vi "Get Next Round.vi"(11 "Square in":refnum<class "Square.lvclass">) -> (2 "Next Round":u32, 3 "Square out":refnum<class "Square.lvclass">)   [LabVIEW 2020, in "SquareBattle.lvlib" / "Square.lvclass"]
uses:
  Square.lvclass
  Square.lvclass/Square.ctl
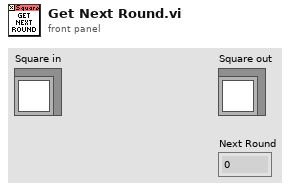
[diagram p1: front panel]
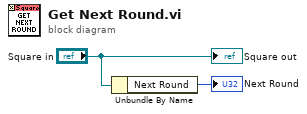
[diagram p0: block diagram]
diagram:
  n1 = Unbundle By Name("Square in") -> ("Next Round"=→"Next Round":u32)
  "Square out" <- "Square in"
